vi "configureForStandardFunction.vi"(2 "error in (no error)":errorcluster, 3 "Output Properties":T1, 4 "AnalogOutput in":refnum<class "AnalogOutput.lvclass">) -> (0 "error out":errorcluster, 1 "AnalogOutput out":refnum<class "AnalogOutput.lvclass">)   [LabVIEW 2011, in "Hardware.lvlib" / "Channels.lvlib" / "AnalogOutput.lvclass"]
uses:
  AnalogOutput.lvclass
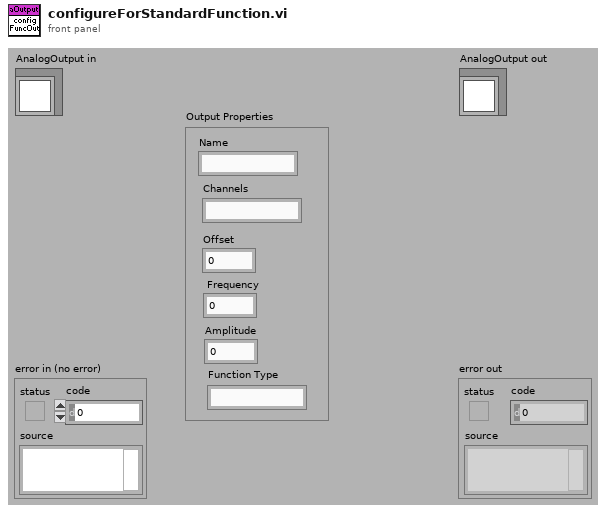
[diagram p1: front panel]
types:
  T1 = cluster{"Name":string, "Channels":string, "Offset":dbl, " Frequency":dbl, "Amplitude":dbl, "Function Type":string}
  T2 = cluster{"Offset":dbl, " Frequency":dbl, "Amplitude":dbl}
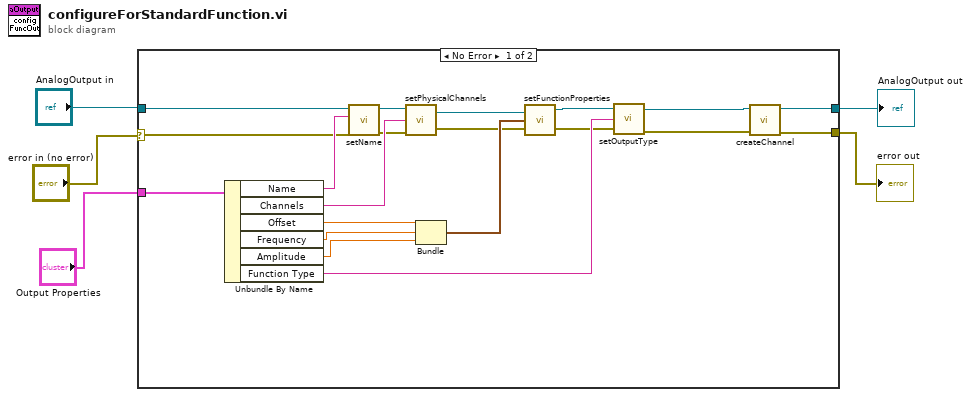
[diagram p0: block diagram]
diagram:
  n1 = case shown="No Error" "error in (no error)" {
    selector: "error in (no error)" -> [w20 w27]
    tunnel: [w19 w27] -> w4
    tunnel: [w18 w26] -> w2
    tunnel: "AnalogOutput in" -> [w21 w26]
    tunnel: "Output Properties" -> [w15 _]
    frame No Error {
      n2 = Unbundle By Name(w15) -> ("Name"=w25:string, "Channels"=w23:string, "Offset"=w14:dbl, "Frequency"=w13:dbl, "Amplitude"=w12:dbl, "Function Type"=w16:string)
      n3 = call "setName.vi"("error in (no error)"=w20, "name"=w25, "AnalogOutput.lvclass in"=w21) -> ("error out"=w22:errorcluster, "AnalogOutput.lvclass out"=w24:refnum<class "AnalogOutput.lvclass">)  [unwired: 7 in]
      n4 = call-dynamic "setPhysicalChannels.vi"("error in (no error)"=w22, "Physical Channels"=w23, "AnalogOutput.lvclass in"=w24) -> ("error out"=w10:errorcluster, "AnalogOutput.lvclass out"=w9:refnum<class "AnalogOutput.lvclass">)
      n5 = Bundle("Offset"=w14, "Frequency"=w13, "Amplitude"=w12) -> (w11:T2)  [unwired: 1 in]
      n6 = call "setFunctionProperties.vi"("error in (no error)"=w10, "Function Properties"=w11, "AnalogOutput in"=w9) -> ("error out"=w7:errorcluster, "AnalogOutput out"=w8:refnum<class "AnalogOutput.lvclass">)
      n7 = call "setOutputType.vi"("error in (no error)"=w7, "Output Type"=w16, "AnalogOutput in"=w8) -> ("error out"=w17:errorcluster, "AnalogOutput out"=w6:refnum<class "AnalogOutput.lvclass">)
      n8 = call-dynamic "createChannel.vi"("error in (no error)"=w17, "AnalogOutput in"=w6) -> ("error out"=w19:errorcluster, "AnalogOutput out"=w18:refnum<class "AnalogOutput.lvclass">)  [unwired: 8 in]
    }
    frame Error {
    }
  }
  "error out" <- w4
  "AnalogOutput out" <- w2
